vi "Many BLM Control Com.vi"() -> (0 "Command text":string[][](array[string]))   [LabVIEW 2020]
uses:
  BLM Control.ctl
panel:
  in  "Initial Distance":dbl
  in  "Final Distance":dbl
  in  "Number of Interval":dbl
  in  "Generate":bool
  in  "cancel":bool
  in  "next":bool
  in  "BLM Control":T1={"extra wait"=0, "Stepper Value"=1.0, "Value 1"=0.0, "Value 2"=1.0, "String 1"="", "String 2"=""} {"Value 2" format="%#_6e"; "Value 1" format="%#_6e"; "extra wait" min=0; "Stepper Value" step=0.045 format="%#.7e"}
  in  "wait after moving (sec)":i32
  out "loop array":dbl[][](array[numeric])
  in  "Array":dbl[][](array[numeric]) format="%#_4e"
  # "BLM (Brushless Motor) Control"
  # "Multiple Input Generator"
  # "(BLM_ManualControl.vi needs to be open before using this program)"
  # "generates multiple BLM values for the sequence, see belolw.  If you like it click \"Good, use this!\". You can also modify the values directly from the following array."
  # "Value"
  # "BLM (Brushless Motor) Control"
  # "(BLM_ManualControl.vi needs to be open before using this program)"
  # "Distance:"
  # "deg of BLM:"
  # "seconds"
  # "AND wait extra"
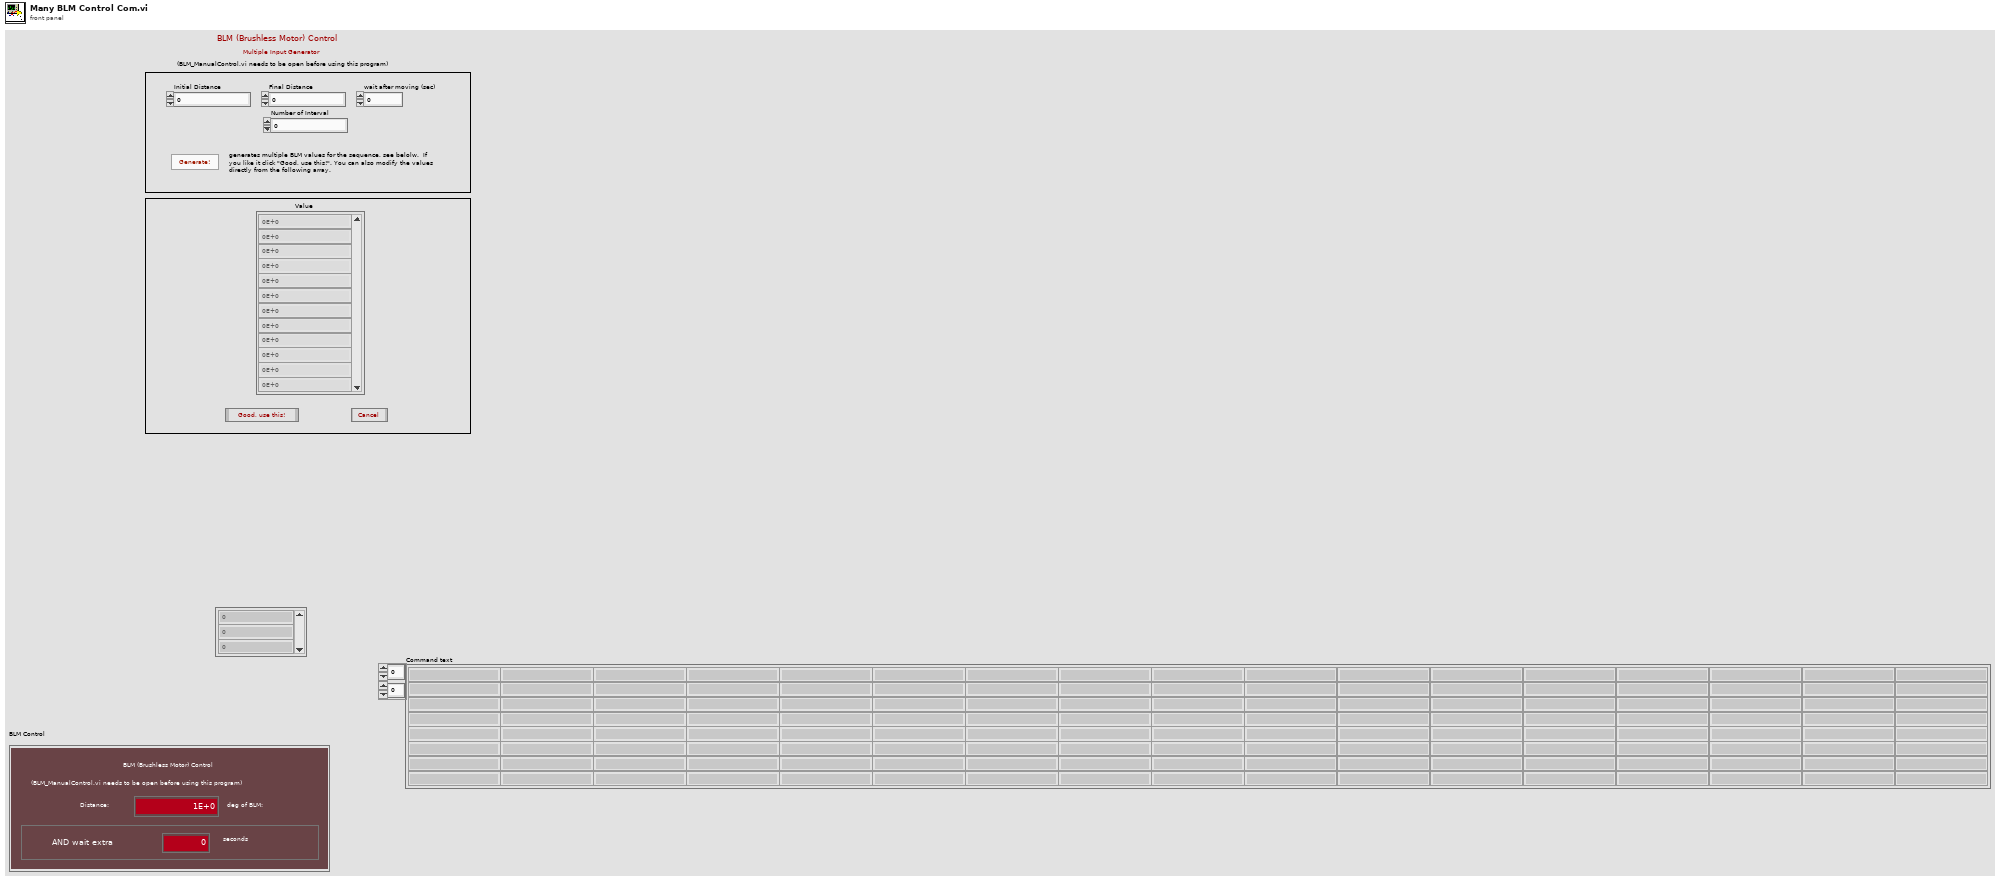
[diagram p1: front panel]
types:
  T1 = typedef "BLM Control.ctl" = cluster{"extra wait":i32, "Stepper Value":dbl, "Value 1":dbl, "Value 2":dbl, "String 1":string, "String 2":string}
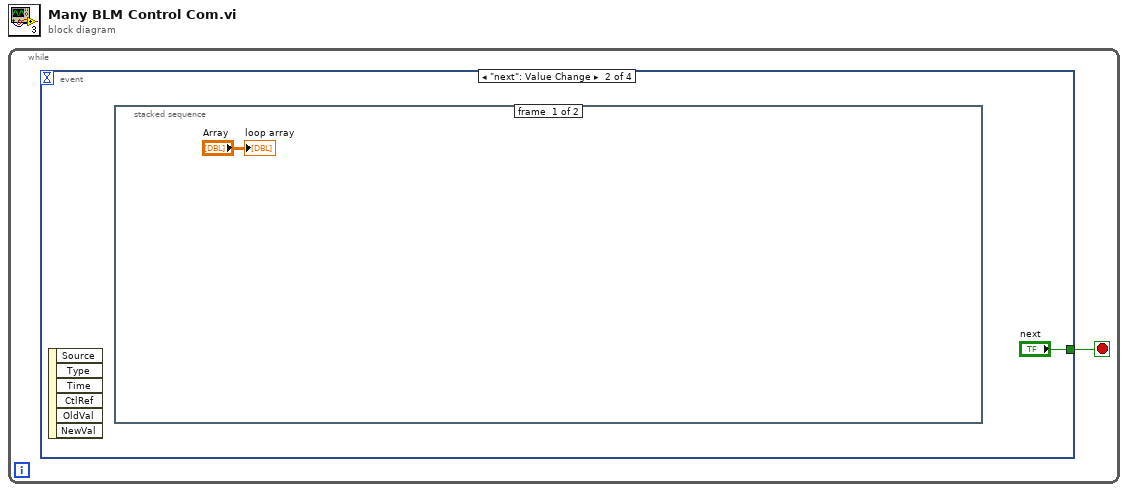
[diagram p0: block diagram]
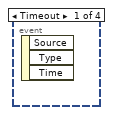
[diagram p2: hidden frame]
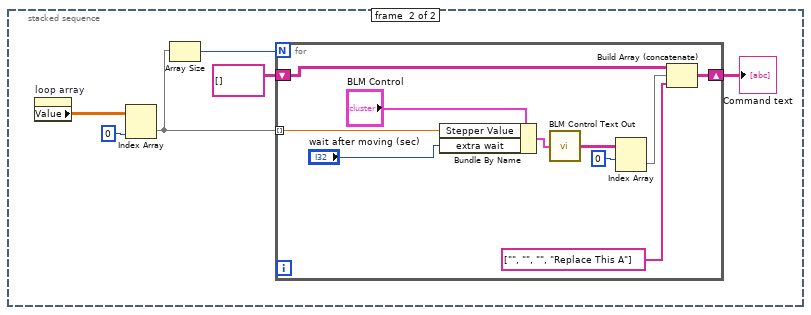
[diagram p3: hidden frame]
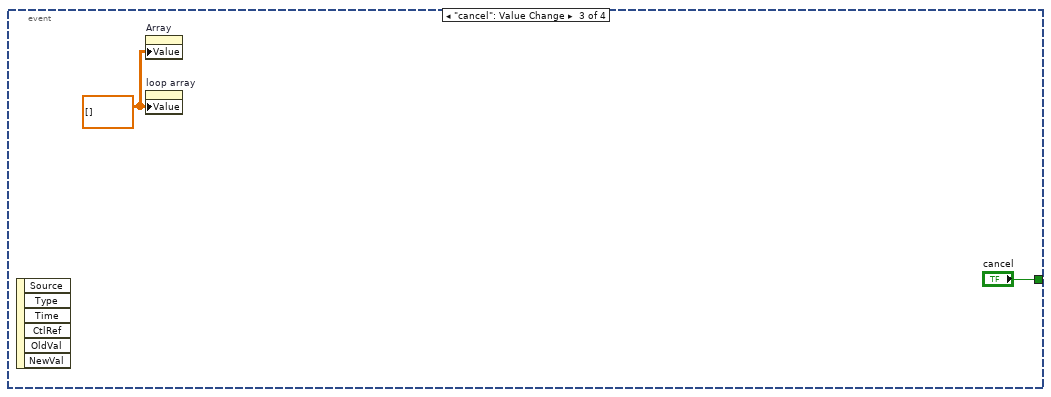
[diagram p4: hidden frame]
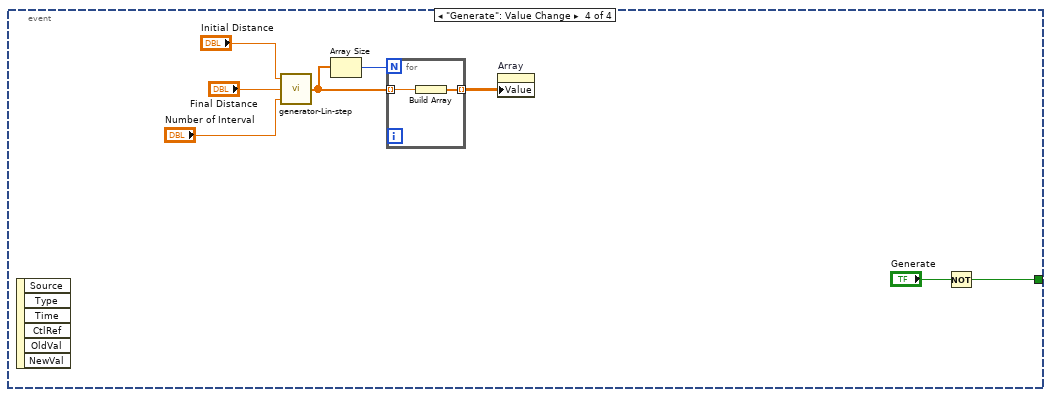
[diagram p5: hidden frame]
diagram:
  n1 = while {
    stop <- w1 stop-if-true
    n2 = event shown="[1] \"next\": Value Change" {
      selector: _ -> [_ _ _ _]
      dyn-events: _ -> [_ _ _ _]
      timeout: _ -> [_ _ _ _]
      tunnel: [_ "next" "cancel" w24] -> w1
      event Timeout {
        n3 = event-data() -> ()  [unwired: 1 in, 3 out]
      }
      event "next": Value Change {
        n4 = event-data() -> ()  [unwired: 1 in, 6 out]
        n5 = stacked-sequence {
          frame #0 {
            "loop array" <- "Array"
          }
          frame #1 {
            n6 = property on="loop array" class="Arr (strict)"() -> ("Value"=w8:dbl[][])  [unwired: 2 in, 2 out]
            n7 = Index Array(array=w8, index (col)=0 ("disabled index (col)")) -> (element=w7:dbl[])  [unwired: 1 in]
            n8 = Array Size(array=w7) -> (size(s)=w6:i32)
            n9 = for {
              N: w6 -> [_]
              tunnel: w7 -> [w11] mode=indexing
              shift-right: [w13] -> w5
              shift-left: string[][] [] -> [w12]
              n10 = Bundle By Name(cluster="BLM Control", "Stepper Value"=w11, "extra wait"="wait after moving (sec)") -> (w10:T1)
              n11 = call "BLM Control Text Out.vi"("BLM Control"=w10) -> ("Command text"=w17:string[][])
              n12 = Index Array(array=w17, index (row)=0) -> (element=w15:string[])  [unwired: 1 in]
              n13 = Build Array (concatenate)(w12, w15, string[] ["", "", "", "Replace This A"]) -> (w13:string[][])
            }
            "Command text" <- w5
          }
        }
      }
      event "cancel": Value Change {
        w20 = dbl[][] [] ("Array")
        n14 = event-data() -> ()  [unwired: 1 in, 6 out]
        n15 = property on="Array" class="Arr (strict)"("Value"=w20) -> ()  [unwired: 2 in, 2 out]
        n16 = property on="loop array" class="Arr (strict)"("Value"=w20) -> ()  [unwired: 2 in, 2 out]
      }
      event "Generate": Value Change {
        n17 = event-data() -> ()  [unwired: 1 in, 6 out]
        n18 = call "generator-Lin-step.vi"("step"="Number of Interval", "end"="Final Distance", "start"="Initial Distance") -> ("Array"=w23:dbl[])
        n19 = Array Size(array=w23) -> (size(s)=w25:i32)
        n20 = for {
          N: w25 -> [_]
          tunnel: w23 -> [w31] mode=indexing
          tunnel: [w30] -> w22 mode=indexing
          n21 = Build Array(w31) -> (w30:dbl[])
        }
        n22 = property on="Array" class="Arr (strict)"("Value"=w22) -> ()  [unwired: 2 in, 2 out]
        n23 = Not(x="Generate") -> (.not. x?=w24:bool)
      }
    }
  }
